vi "Close.vi"(8 "error in (no error)":errorcluster, 11 "LXIPXISwitching in":refnum<class "LXIPXISwitching.lvclass">) -> (0 "error out":errorcluster, 3 "LXIPXISwitching out":refnum<class "LXIPXISwitching.lvclass">)   [LabVIEW 2018, in "LXIPXISwitching.lvclass"]
uses:
  LXIPXISwitching.lvclass
  LXIPXISwitching.lvclass/LXIPXISwitching.ctl
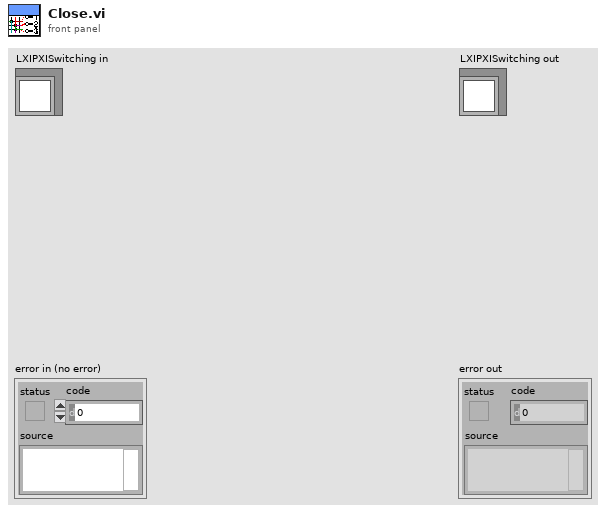
[diagram p1: front panel]
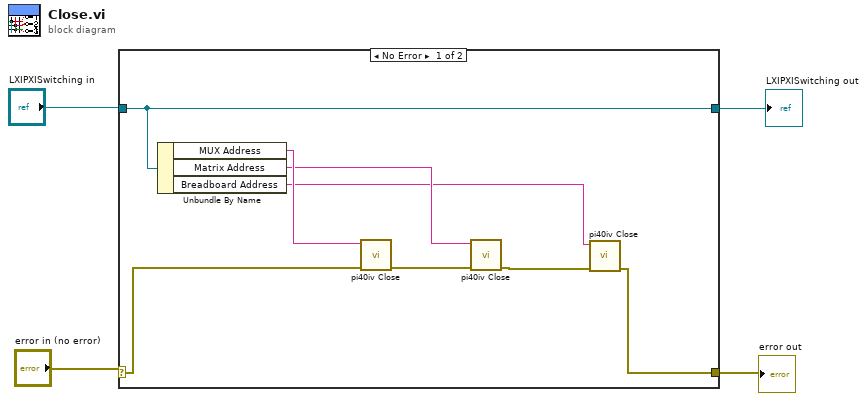
[diagram p0: block diagram]
diagram:
  n1 = case shown="No Error" "error in (no error)" {
    selector: "error in (no error)" -> [w12 w14]
    tunnel: [w9 w14] -> w3
    tunnel: [w8 w13] -> w1
    tunnel: "LXIPXISwitching in" -> [w8 w13]
    frame No Error {
      n2 = Unbundle By Name(w8) -> ("MUX Address"=w7:string, "Matrix Address"=w6:string, "Breadboard Address"=w5:string)
      n3 = call <instrlib>:"pi40iv Close.vi"("error in (no error)"=w12, "instrument handle"=w7) -> ("error out"=w11:errorcluster)  [unwired: 9 in]
      n4 = call <instrlib>:"pi40iv Close.vi"("error in (no error)"=w11, "instrument handle"=w6) -> ("error out"=w10:errorcluster)  [unwired: 9 in]
      n5 = call <instrlib>:"pi40iv Close.vi"("error in (no error)"=w10, "instrument handle"=w5) -> ("error out"=w9:errorcluster)  [unwired: 9 in]
    }
    frame Error {
    }
  }
  "error out" <- w3
  "LXIPXISwitching out" <- w1
